vi "Write TestRole 1.vi"(8 "error in (no error)":errorcluster, 10 "TestRole":refnum<class "TestRole.lvclass">, 11 "TestPlay in":refnum<class "TestPlay.lvclass">) -> (0 "error out":errorcluster, 3 "TestPlay out":refnum<class "TestPlay.lvclass">)   [LabVIEW 2023, in "TestPlay.lvclass"]
uses:
  TestPlay.lvclass
  TestRole_class/TestRole.lvclass
  TestPlay.lvclass/TestPlay.ctl
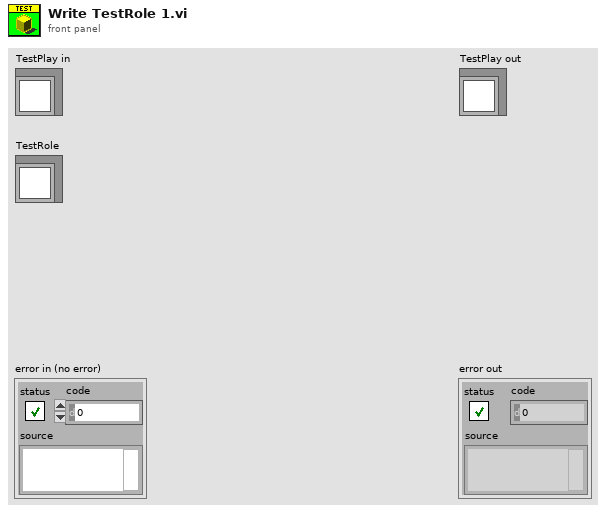
[diagram p1: front panel]
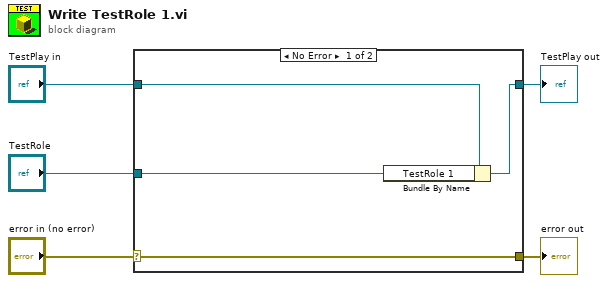
[diagram p0: block diagram]
diagram:
  n1 = case shown="No Error" "error in (no error)" {
    selector: "error in (no error)" -> [w9 w10]
    tunnel: [w9 w10] -> w4
    tunnel: [w7 w11] -> w2
    tunnel: "TestPlay in" -> [w8 w11]
    tunnel: "TestRole" -> [w6 _]
    frame No Error {
      n2 = Bundle By Name(cluster=w8, "TestRole 1"=w6) -> (w7:refnum<class "TestPlay.lvclass">)
    }
    frame Error {
    }
  }
  "error out" <- w4
  "TestPlay out" <- w2
